vi "Create Channel Waveform.vi"(6 "Channel index":i32, 8 "error in (no error)":errorcluster, 10 "Data":i16[](array[numeric]), 11 "Red Pitaya Digitizer in":refnum<class "Red Pitaya Digitizer.lvclass">) -> (0 "error out":errorcluster, 1 "Waveform out":waveform(i16), 3 "Red Pitaya Digitizer out":refnum<class "Red Pitaya Digitizer.lvclass">)   [LabVIEW 2015, in "Red Pitaya Digitizer.lvclass"]
uses:
  Red Pitaya Digitizer.lvclass
  Red Pitaya Digitizer.lvclass/Red Pitaya Digitizer.ctl
  Instruments/Pulse Driver/Pulse Driver.lvclass
  RP Core/RP Instrument/RP Instrument.lvclass
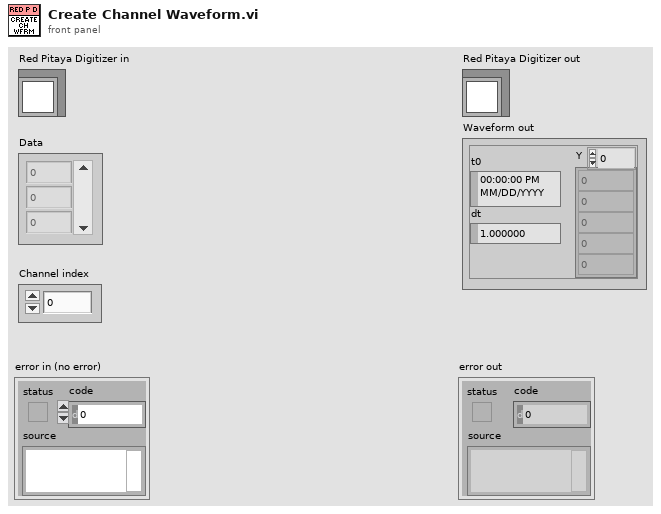
[diagram p1: front panel]
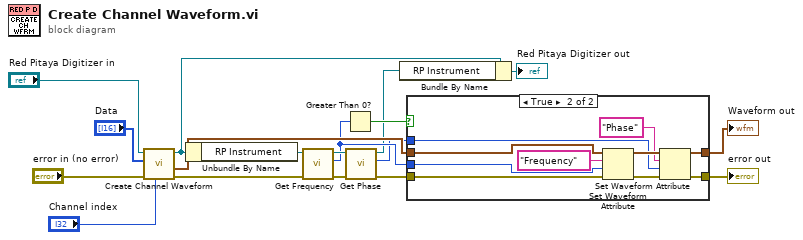
[diagram p0: block diagram]
diagram:
  n1 = call-parent "Create Channel Waveform.vi"("Channel index"="Channel index", "error in (no error)"="error in (no error)", "Data"="Data", "Pulse Driver in"="Red Pitaya Digitizer in") -> ("error out"=w3:errorcluster, "Waveform out"=w10:waveform(i16), "Pulse Driver out"=w14:refnum<class "Red Pitaya Digitizer.lvclass">)  [unwired: 5 in]
  n2 = Unbundle By Name(w14) -> ("RP Instrument"=w13:refnum<class "RP Instrument.lvclass">)
  n3 = call-dynamic "Get Frequency.vi"("error in (no error)"=w3, "RP Instrument in"=w13) -> ("error out"=w12:errorcluster, "Frequency"=w7:u32, "RP Instrument out"=w11:refnum<class "RP Instrument.lvclass">)  [unwired: 7 in]
  n4 = Greater Than 0?(x=w7) -> (x > 0?=w8:bool)
  n5 = call-dynamic "Get Phase.vi"("error in (no error)"=w12, "RP Instrument in"=w11) -> ("error out"=w9:errorcluster, "Phase"=w6:u32, "RP Instrument out"=w4:refnum<class "RP Instrument.lvclass">)  [unwired: 7 in]
  n6 = Bundle By Name(cluster=w14, "RP Instrument"=w4) -> (→"Red Pitaya Digitizer out":refnum<class "Red Pitaya Digitizer.lvclass">)
  n7 = case shown="True" w8 {
    tunnel: w10 -> [w19 w30]
    tunnel: [w19 w28] -> w1
    tunnel: [w20 w27] -> w2
    tunnel: w9 -> [w20 w26]
    tunnel: w7 -> [_ w23]
    tunnel: w6 -> [_ w21]
    frame False {
    }
    frame True {
      n8 = Set Waveform Attribute(4:w26, 5:w23, 6:"Frequency" ("name"), 7:w30) -> (0:w25:errorcluster, 3:w29:waveform(i16))  [unwired: 1 out]
      n9 = Set Waveform Attribute(4:w25, 5:w21, 6:"Phase" ("name"), 7:w29) -> (0:w27:errorcluster, 3:w28:waveform(i16))  [unwired: 1 out]
    }
  }
  "error out" <- w2
  "Waveform out" <- w1
